vi "Rtn Freq Cal Para.vi"(7 "capValue":u32, 8 "error in (no error)":errorcluster, 9 "iNumAvg":u32, 10 "dPowerLevel":dbl, 11 "iFreq":u32) -> (0 "error out":errorcluster, 1 "iNumAvg out":u32, 2 "dPowerLevel out":dbl, 3 "iFreq out":u32, 5 "capValue out":u32)   [LabVIEW 2013, in "QCAWLAN_DLL.lvlib"]
doc: "QCA_DLL_Export void RtnFreqCalPara(unsigned int* iFreq, double* dPowerLevel, unsigned int* iNumAvg, unsigned int* capValue);"
uses:
  QCAWLAN_DLL.lvlib
  QCAWLAN_DLL.dll
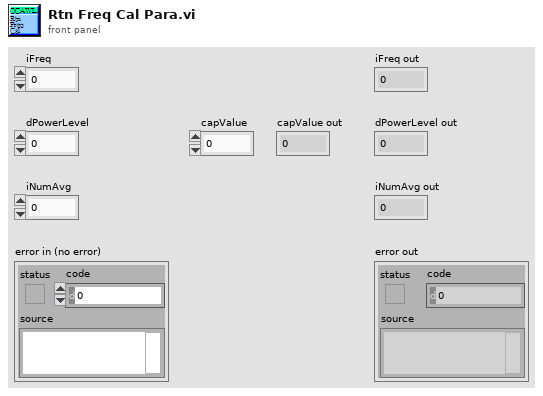
[diagram p1: front panel]
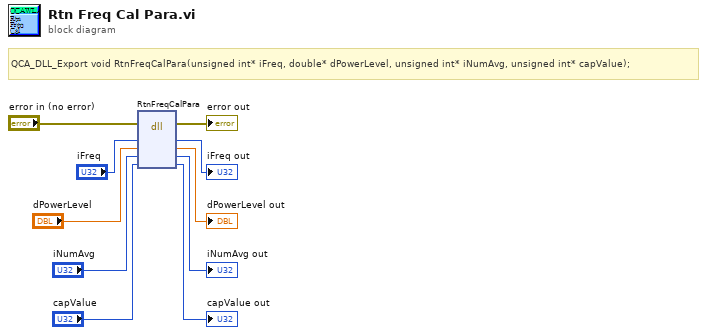
[diagram p0: block diagram]
diagram:
  # "QCA_DLL_Export void RtnFreqCalPara(unsigned int* iFreq, double* dPowerLevel, unsigned int* iNumAvg, unsigned int* capValue);"
  n1 = dll-call lib="C:/Connectivity Client - MIMO/PlugIn/QCAWLAN_DLL.*" fn="RtnFreqCalPara"(error in="error in (no error)", "iFreq"="iFreq", "dPowerLevel"="dPowerLevel", "iNumAvg"="iNumAvg", "capValue"="capValue") -> (error out=→"error out":errorcluster, "iFreq"=→"iFreq out":u32, "dPowerLevel"=→"dPowerLevel out":dbl, "iNumAvg"=→"iNumAvg out":u32, "capValue"=→"capValue out":u32)  [unwired: 3 in, 1 out]
